vi "string numbers in range.vi"(8 "error in (no error)":errorcluster, 9 "String 2":string, 10 "String":string, 11 "tolerance":dbl) -> (0 "error out":errorcluster, 3 "Boolean":bool)   [LabVIEW 2020]
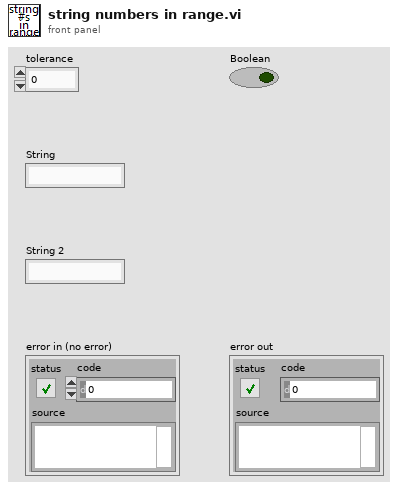
[diagram p1: front panel]
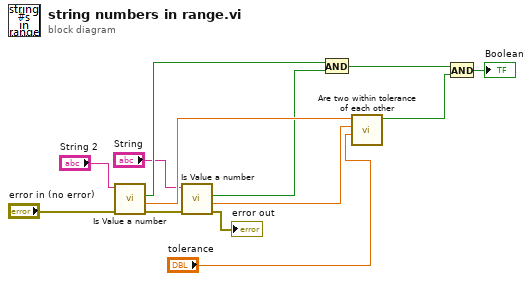
[diagram p0: block diagram]
diagram:
  n1 = call "Is Value a number.vi"("user error in"="error in (no error)", "value String"="String 2") -> ("user error out"=w6:errorcluster, "number"=w9:dbl, "a number"=w3:bool)  [unwired: 6 in, 1 out]
  n2 = call "Is Value a number.vi"("user error in"=w6, "value String"="String") -> ("user error out"=→"error out":errorcluster, "number"=w10:dbl, "a number"=w4:bool)  [unwired: 6 in, 1 out]
  n3 = And(x=w3, y=w4) -> (x .and. y?=w5:bool)
  n4 = call "Are two within tolerance of each other.vi"("tolerance"="tolerance", "number 2"=w10, "number"=w9) -> ("In range"=w13:bool)  [unwired: 8 in]
  n5 = And(x=w5, y=w13) -> (x .and. y?=→"Boolean":bool)
